vi "morse.vi"() -> ()   [LabVIEW 2015]
panel:
  out "Morse out":string
  in  "String in":string
  in  "dot time":u32
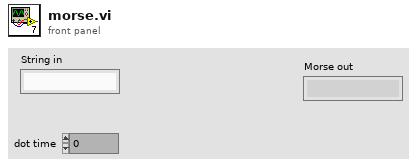
[diagram p1: front panel]
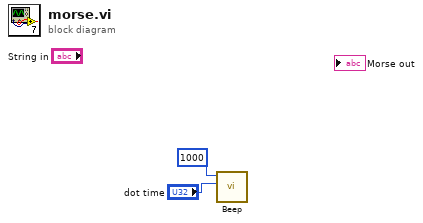
[diagram p0: block diagram]
diagram:
  n1 = call <vilib>:"Beep.vi"("duration (msec)"="dot time", "frequency (Hz)"=u32 1000) -> ()  [unwired: 10 in]
